vi "ListLibraryFolders.vi"(11 "Path":path) -> (2 "All Folders":path[](array[path]), 3 "Include List":string)   [LabVIEW 2010]
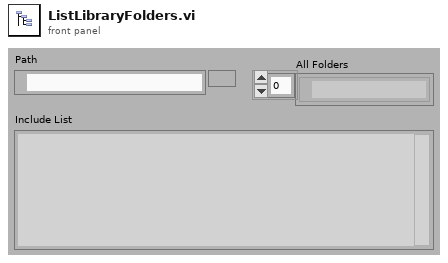
[diagram p1: front panel]
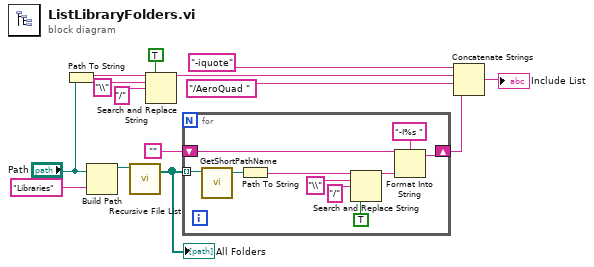
[diagram p0: block diagram]
diagram:
  n1 = Path To String(path="Path") -> (string=w9:string)
  n2 = Build Path(base path="Path", name or relative path="Libraries") -> (appended path=w13:path)
  n3 = call <vilib>:"Recursive File List.vi"("Folder Path"=w13) -> ("All Folders"=w1:path[])  [unwired: 6 in, 4 out]
  "All Folders" <- w1
  n4 = Search and Replace String(replace all?=TRUE ("replace all? (F)"), input string=w9, search string="\\", replace string="/" ("replace string (\"\")")) -> (result string=w5:string)  [unwired: 4 in, 3 out]
  n5 = for {
    shift-right: [w23] -> w3
    shift-left: "" -> [w24]
    tunnel: w1 -> [w17] mode=indexing
    n6 = call "GetShortPathName.vi"("Long Path In:"=w17) -> ("Short Path Out:"=w16:path)  [unwired: 8 in, 2 out]
    n7 = Path To String(path=w16) -> (string=w15:string)
    n8 = Search and Replace String(replace all?=TRUE ("replace all? (F)"), input string=w15, search string="\\", replace string="/" ("replace string (\"\")")) -> (result string=w18:string)  [unwired: 4 in, 3 out]
    n9 = Format Into String(format string="-I%s ", initial string=w24, w18) -> (resulting string=w23:string)  [unwired: 1 in, 1 out]
  }
  n10 = Concatenate Strings("-iquote" ("string"), w5, "/AeroQuad " ("name or relative path"), w3) -> (→"Include List":string)
